vi "Controller Process.vi"(8 "error in (no error)":errorcluster, 11 "View Model":T1) -> (0 "error out":errorcluster)   [LabVIEW 2017]
uses:
  View Model/Controls/View Model.ctl
  Configuration Database/Controls/Config Model.ctl
  Configuration Database/Controls/Config Commands.ctl
  Configuration Database/Controls/Congif Data.ctl
  View Model/Controls/Shared Model.ctl
  Error Handler/Controls/Error Model.ctl
  Error Handler/Controls/Error Data.ctl
  Error Handler/Controls/Error Type.ctl
  Controls/Car Wash Model.ctl
  Controls/Controller Overhead.ctl
  Controls/Vehicle Location.ctl
  Controls/Car Wash States.ctl
  Controls/CarWash CMD.ctl
  Views/Wash Display Console View/Controls/Car Wash Indicators.ctl
  Views/Entry Console View/Controls/Entry Console Data.ctl
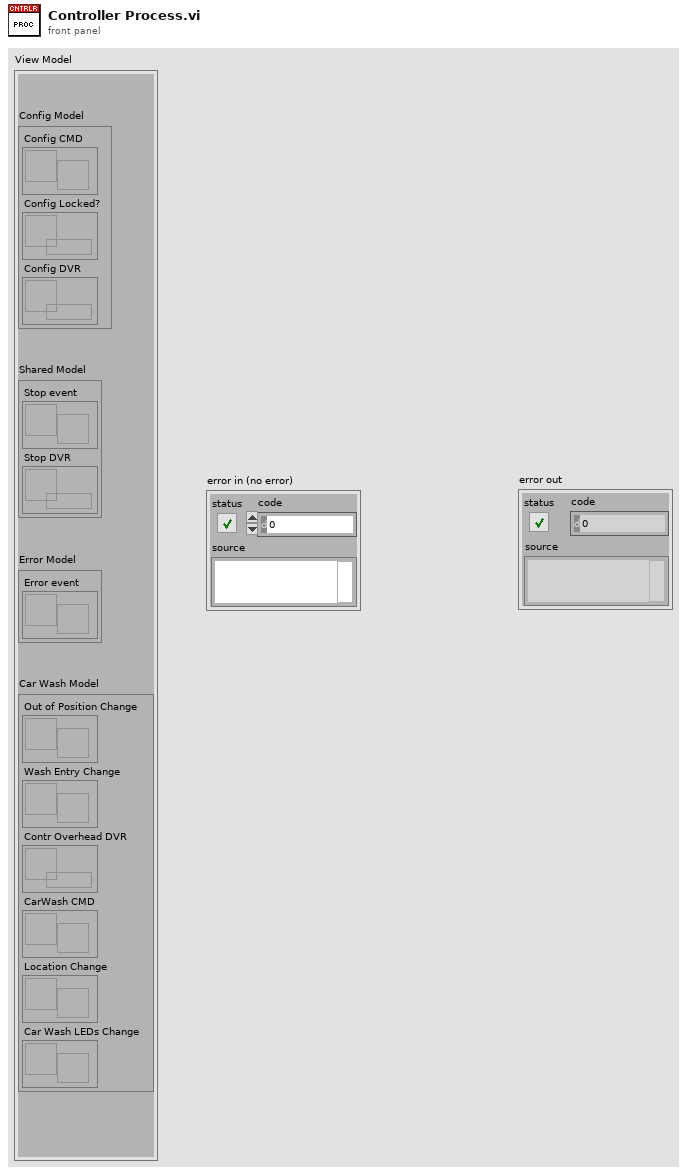
[diagram p1: front panel]
types:
  T1 = typedef "View Model.ctl" = cluster{"Config Model":T2, "Shared Model":T3, "Error Model":T4, "Car Wash Model":T5}
  T2 = typedef "Config Model.ctl" = cluster{"Config CMD":refnum<user-event>, "Config Locked?":refnum<data-value>, "Config DVR":refnum<data-value>}
  T3 = typedef "Shared Model.ctl" = cluster{"Stop event":refnum<user-event>, "Stop DVR":refnum<data-value>}
  T4 = typedef "Error Model.ctl" = cluster{"Error event":refnum<user-event>}
  T5 = typedef "Car Wash Model.ctl" = cluster{"Out of Position Change":refnum<user-event>, "Wash Entry Change":refnum<user-event>, "Contr Overhead DVR":refnum<data-value>, "CarWash CMD":refnum<user-event>, "Location Change":refnum<user-event>, "Car Wash LEDs Change":refnum<user-event>}
  T6 = typedef "Entry Console Data.ctl" = cluster{"Under Body Wash":bool, "Bug Remover":bool, "Pre-Soak":bool, "High Pressure Wash":bool, "Low Pressure Wax":bool, "Spot Free Rinse":bool, "Tire Shine Foam":bool, "Air Dry":bool}
  T7 = typedef "Config Commands.ctl" = enum16{"Read records", "Query timing data", "Insert new data records", "Update data records"}
  T8 = typedef "Car Wash States.ctl" = enum16{"Initial", "Wait for start", "Start", "Wait for vehicle", "Wash Step Execution", "Wash Step/Cycle Complete", "Wash Exit", "Wash Abort/Terminate"}
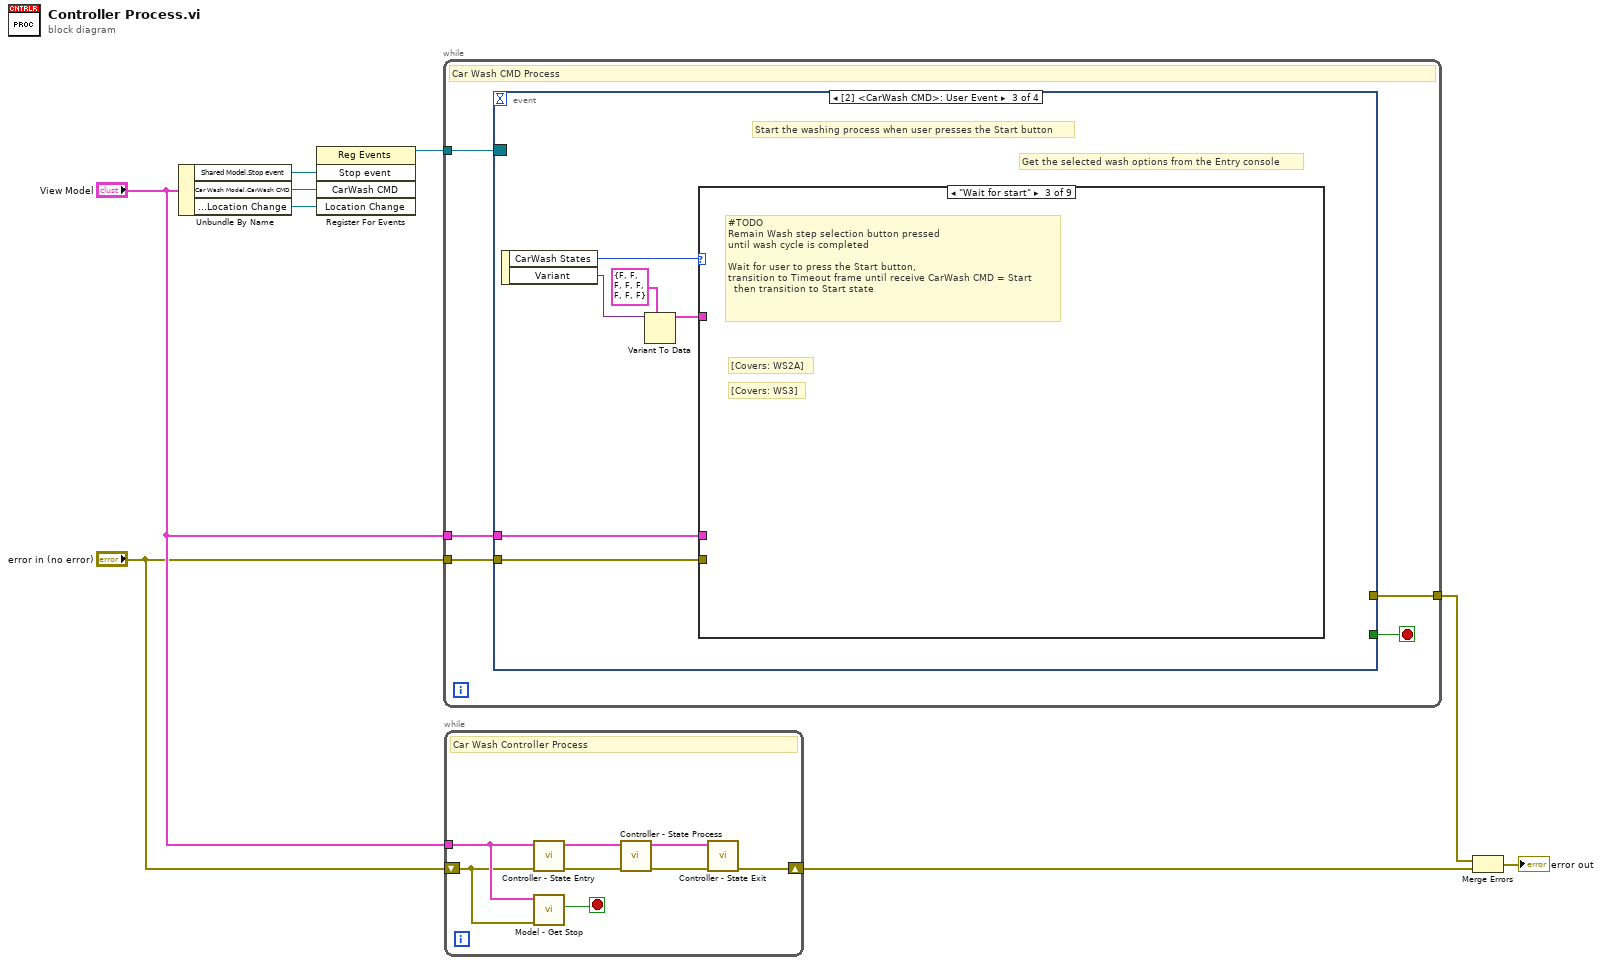
[diagram p0: block diagram]
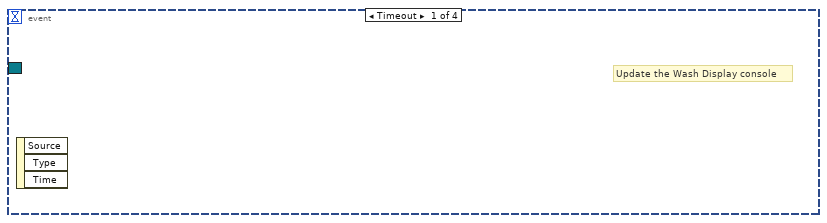
[diagram p2: hidden frame]
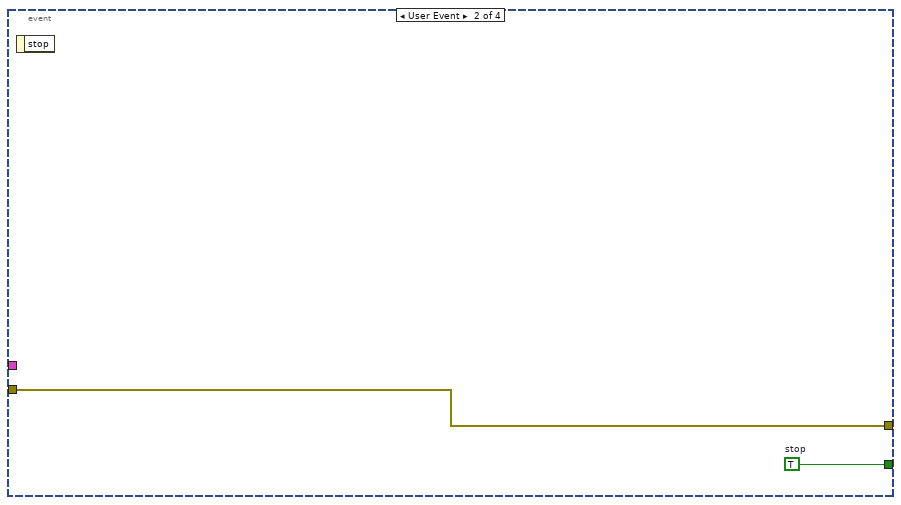
[diagram p3: hidden frame]
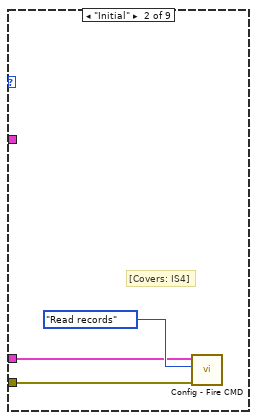
[diagram p5: hidden frame]
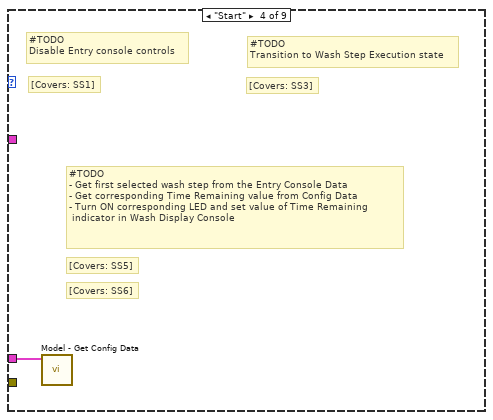
[diagram p6: hidden frame]
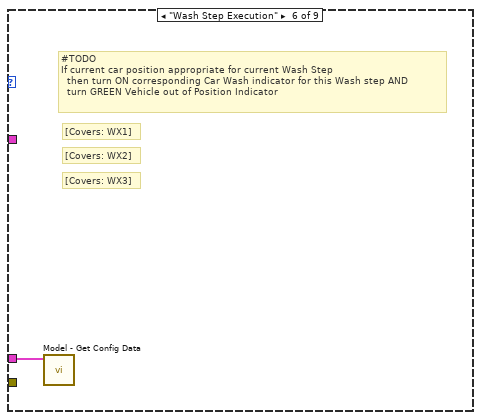
[diagram p8: hidden frame]
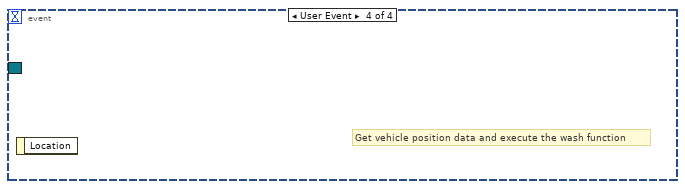
[diagram p12: hidden frame]
diagram:
  n1 = Unbundle By Name("View Model") -> ("Shared Model.Stop event"=w9:refnum<user-event>, "Car Wash Model.CarWash CMD"=w7:refnum<user-event>, "Car Wash Model.Location Change"=w6:refnum<user-event>)
  n2 = register-events(w9, w7, w6) -> (reference out=w8:refnum<event-registration>)  [unwired: 2 in, 1 out]
  n3 = while {
    tunnel: w8 -> [w14]
    tunnel: "error in (no error)" -> [w12]
    tunnel: [w11] -> w3
    tunnel: "View Model" -> [w10]
    stop <- w13 stop-if-true
    # "Car Wash CMD Process"
    n4 = event shown="[2] <CarWash CMD>: User Event" {
      selector: w14 -> [_ _ _ _]
      dyn-events: _ -> [_ _ _ _]
      timeout: _ -> [_ _ _ _]
      tunnel: [_ w16 _ _] -> w13
      tunnel: w12 -> [_ w15 w17 _]
      tunnel: [_ w15 _ _] -> w11
      tunnel: w10 -> [_ _ w18 _]
      event Timeout {
        # "Update the Wash Display console"
        n5 = event-data() -> ()  [unwired: 1 in, 3 out]
      }
      event User Event {
        w16 = TRUE  # stop
        n6 = event-data() -> ()  [unwired: 1 in, 1 out]
      }
      event User Event {
        # "Get the selected wash options from the Entry console"
        # "Start the washing process when user presses the Start button"
        n7 = event-data() -> ("CarWash States"=w22:T8, "Variant"=w20:variant)  [unwired: 1 in]
        n8 = Variant To Data(type=T6 {"Under Body Wash"=FALSE, "Bug Remover"=FALSE, "Pre-Soak"=FALSE, "High Pressure Wash"=FALSE, "Low Pressure Wax"=FALSE, "Spot Free Rinse"=FALSE, "Tire Shine Foam"=FALSE, "Air Dry"=FALSE} ("Entry Console Data"), Variant=w20) -> (data=w19:T6)  [unwired: 1 in, 1 out]
        n9 = case shown="\"Wait for start\"" w22 {
          tunnel: w19 -> [_ _ _ _ _ _ _ _ _]
          tunnel: w18 -> [_ w24 _ w26 _ w27 _ _ _]
          tunnel: w17 -> [_ w23 _ _ _ _ _ _ _]
          frame Default {
          }
          frame "Initial" {
            # "[Covers: IS4]"
            n10 = call "Config - Fire CMD.vi"("error in (no error)"=w23, "Config CMD"=Config_Commands."Read records", "View Model"=w24) -> ()  [unwired: 7 in, 2 out]
          }
          frame "Wait for start" {
            # "[Covers: WS3]"
            # "[Covers: WS2A]"
            # "#TODO\nRemain Wash step selection button pressed\nuntil wash cycle is completed\n\nWait for user to press the Start button, \ntransition to Timeout frame until receive CarWash CMD = Start\n  then transition to Start state"
          }
          frame "Start" {
            # "[Covers: SS6]"
            # "[Covers: SS5]"
            # "#TODO\n- Get first selected wash step from the Entry Console Data\n- Get corresponding Time Remaining value from Config Data\n- Turn ON corresponding LED and set value of Time Remaining\n indicator in Wash Display Console"
            # "[Covers: SS3]"
            # "#TODO\nTransition to Wash Step Execution state"
            # "[Covers: SS1]"
            # "#TODO\nDisable Entry console controls"
            n11 = call "Model - Get Config Data.vi"("View Model"=w26) -> ()  [unwired: 8 in, 3 out]
          }
          frame "Wait for vehicle" {
            # "[Covers: VS4]"
            # "#TODO\nWait untile user move the car to corresponding for active Wash step position.\nIf active step is last then wait for car moves to Exit"
            # "[Covers: VS3]"
            # "[Covers: VS2]"
            # "[Covers: VS1]"
            # "#TODO\n- Turn ON Car Wash indicator in accordance to active Wash Step\n- Turn RED Vehicle out of Position LED\n- Update Time Remaining indicator for the active Wash step's time"
          }
          frame "Wash Step Execution" {
            # "[Covers: WX3]"
            # "[Covers: WX2]"
            # "[Covers: WX1]"
            # "#TODO\nIf current car position appropriate for current Wash Step\n  then turn ON corresponding Car Wash indicator for this Wash step AND\n  turn GREEN Vehicle out of Position Indicator"
            n12 = call "Model - Get Config Data.vi"("View Model"=w27) -> ()  [unwired: 8 in, 3 out]
          }
          frame "Wash Step/Cycle Complete" {
            # "[Covers: WC3C]"
            # "[Covers: WC3B]"
            # "[Covers: WC3A]"
            # "[Covers: WC2C]"
            # "[Covers: WC2B]"
            # "[Covers: WC2A]"
            # "[Covers: WC3]"
            # "[Covers: WC2]"
            # "#TODO\nTurn RED Vehicle out of Position indicator;\nIf the completed wash step was last\nthen -Turn OFF all Car wash indicators\n  - Wait until user move car position to Exit\nelse\n  - Turn on next Car Wash indicator corresponding\n     to next wash step\n  - Wait until user move car to the appropriate station"
            # "[Covers: WC1]"
            # "#TODO\nTurn Off Car Wash indicator correspomding to\ncompleted wash step"
          }
          frame "Wash Exit" {
            # "[Covers: WE4]"
            # "[Covers: WE3]"
            # "[Covers: WE2]"
            # "[Covers: WE1]"
            # "#TODO\n-Turn OFF all Car wash indicators\n- Wait until user move car position to Exit AND\n   reposition vehicle to the Entry position\n- Transition to Initial state"
            # "[Covers: WS2A]"
            # "#TODO\nRelease pressed wash step buttons"
          }
          frame "Wash Abort/Terminate" {
            # "[Covers: TS6]"
            # "[Covers: TS5]"
            # "[Covers: TS4]"
            # "[Covers: TS3]"
            # "[Covers: TS2]"
            # "[Covers: TS1]"
            # "#TODO\n- Disable all components of the Entry Console\n- Abort current executing step (stop event)\n- Turn OFF all Car Wash indicators\n- Turn RED Vehicle out of Position indicator\n- Set Time Remaining indicator to value 0.0\n- Display to user Error Dialog message to move car to the Exit"
          }
        }
      }
      event User Event {
        # "Get vehicle position data and execute the wash function"
        n13 = event-data() -> ()  [unwired: 1 in, 1 out]
      }
    }
  }
  n14 = while {
    tunnel: "View Model" -> [w34]
    shift-right: [w28] -> w4
    shift-left: "error in (no error)" -> [w33]
    stop <- w35 stop-if-true
    # "Car Wash Controller Process"
    n15 = call "Controller - State Entry.vi"("error in (no error)"=w33, "View Model"=w34) -> ("error out"=w32:errorcluster, "View Model"=w31:T1)  [unwired: 8 in]
    n16 = call "Model - Get Stop.vi"("error in (no error)"=w33, "View Model"=w34) -> ("Stop"=w35:bool)  [unwired: 7 in, 2 out]
    n17 = call "Controller - State Process.vi"("error in (no error)"=w32, "View Model"=w31) -> ("error out"=w29:errorcluster, "View Model"=w30:T1)  [unwired: 8 in]
    n18 = call "Controller - State Exit.vi"("error in (no error)"=w29, "View Model"=w30) -> ("error out"=w28:errorcluster)  [unwired: 8 in, 1 out]
  }
  n19 = Merge Errors(w3, w4) -> (→"error out":errorcluster)
